vi "Set Value.vi"(8 "error in (no error)":errorcluster, 10 "Project Info Value":string, 11 "Ring Item Configuration in":refnum<class "Ring Item Configuration.lvclass">) -> (0 "error out":errorcluster, 3 "Ring Item Configuration out":refnum<class "Ring Item Configuration.lvclass">)   [LabVIEW 2013, in "Item Configuration.lvlib" / "Ring Item Configuration.lvclass"]
uses:
  Ring Item Configuration.lvclass
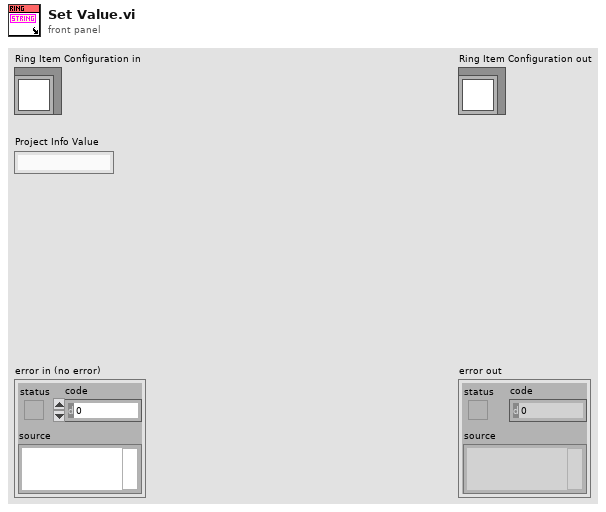
[diagram p1: front panel]
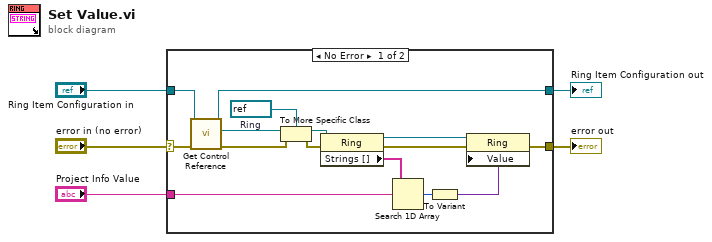
[diagram p0: block diagram]
diagram:
  n1 = case shown="No Error" "error in (no error)" {
    selector: "error in (no error)" -> [w19 w22]
    tunnel: "Ring Item Configuration in" -> [w20 w21]
    tunnel: "Project Info Value" -> [w12 _]
    tunnel: [w7 w22] -> w2
    tunnel: [w6 w21] -> w1
    frame No Error {
      w17 = refnum<vi> refnum  # Ring
      n2 = call-dynamic "Get Control Reference.vi"("error in (no error)"=w19, "Item Configuration in"=w20) -> ("error out"=w16:errorcluster, "Control Reference"=w18:refnum<vi>, "Item Configuration out"=w6:refnum<class "Ring Item Configuration.lvclass">)  [unwired: 7 in]
      n3 = To More Specific Class(target class=w17, reference=w18, error in=w16) -> (specific class reference=w14:refnum<vi>, error out=w15:errorcluster)
      n4 = property class="Ring"(reference=w14, error in=w15) -> (reference out=w8:refnum<vi>, error out=w9:errorcluster, "Strings []"=w13:string[])
      n5 = Search 1D Array(1D array=w13, element=w12) -> (index of element=w11:i32)  [unwired: 1 in]
      n6 = To Variant(anything=w11) -> (Variant=w10:variant)
      n7 = property class="Ring"(reference=w8, error in=w9, "Value"=w10) -> (error out=w7:errorcluster)  [unwired: 1 out]
    }
    frame Error {
    }
  }
  "error out" <- w2
  "Ring Item Configuration out" <- w1
